vi "PROJECT_Layout-VI.vi"() -> ()   [LabVIEW 2022 SP3, in "Project.lvlib"]
doc: "This is the default layout VI for the HSE UI Framework. It features three areas:\n- header (contains the \"SP_Header\" subpanel)\n- navigation (contains the \"SP_Navigation\" subpanel)\n- content (contains the \"SP_Content\" subpanel)\n\nThis VI is loaded by the UI Manager module, the subpanels are then populated with DQMH modules as configured in the UI Manager's configuration file.\n\n____\nHAMPEL SOFTWARE ENGINEERING v2.6.0 (2023-12-19 10:54)"
uses:
  Project.lvlib
panel:
  out "STR_Title":string
  out "PIC_Logo":picture
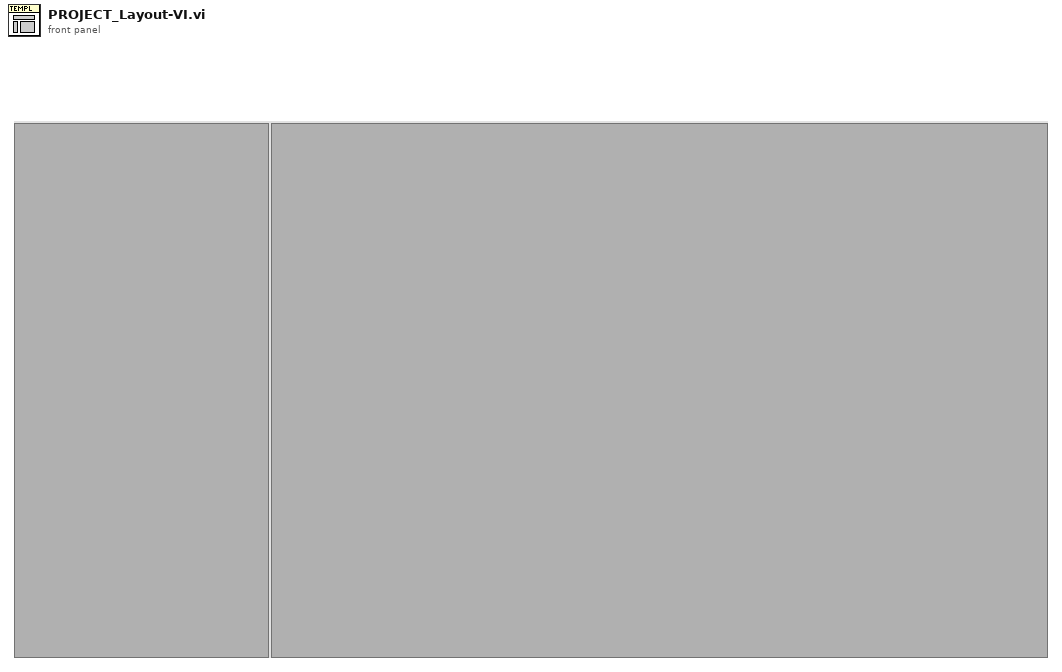
[diagram p1: front panel]
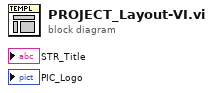
[diagram p0: block diagram]
diagram:
